vi "Write PmuConfig.vi"(8 "error in (no error)":errorcluster, 10 "PmuConfig":T1={"Class"=enum."M", "Fs"=60, "F0"=60, "FSamp"=60, "SettlingTime"=0.0, "T0"=0.0}, 11 "PmuBase in":refnum<class "PmuBase.lvclass">) -> (0 "error out":errorcluster, 3 "PmuBase out":refnum<class "PmuBase.lvclass">)   [LabVIEW 2014, in "SensorPlugins.lvlib" / "PmuBase.lvclass"]
uses:
  PmuBase.lvclass
  Typedef/PmuConfig.ctl
  PmuBase.lvclass/PmuBase.ctl
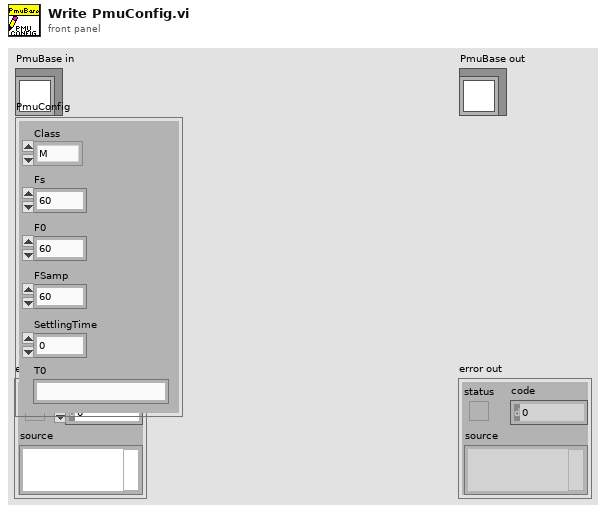
[diagram p1: front panel]
types:
  T1 = typedef "SensorPlugins.lvlib/PmuBase.lvclass/PmuConfig.ctl" = cluster{"Class":enum16{"M", "P"}, "Fs":i32, "F0":i32, "FSamp":i32, "SettlingTime":dbl, "T0":ext}
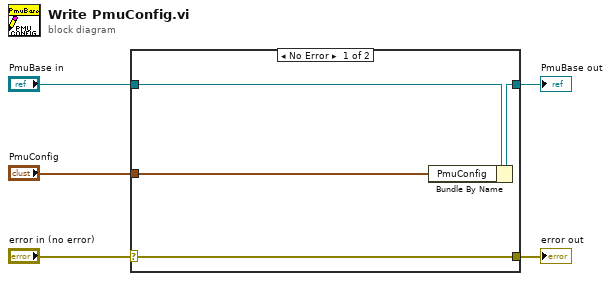
[diagram p0: block diagram]
diagram:
  n1 = case shown="No Error" "error in (no error)" {
    selector: "error in (no error)" -> [w9 w10]
    tunnel: [w9 w10] -> w4
    tunnel: [w7 w11] -> w2
    tunnel: "PmuBase in" -> [w8 w11]
    tunnel: "PmuConfig" -> [w6 _]
    frame No Error {
      n2 = Bundle By Name(cluster=w8, "PmuConfig"=w6) -> (w7:refnum<class "PmuBase.lvclass">)
    }
    frame Error {
    }
  }
  "error out" <- w4
  "PmuBase out" <- w2
